vi "Initialize_Labjacks.vi"() -> (0 "error out":errorcluster, 3 "LJ Handles":i32[](array[numeric])=[546668496, 310679472, 546668496])   [LabVIEW 2016]
uses:
  Globals/LJ_Handles_Global.vi
panel:
  in  "Num Devices":i32=3
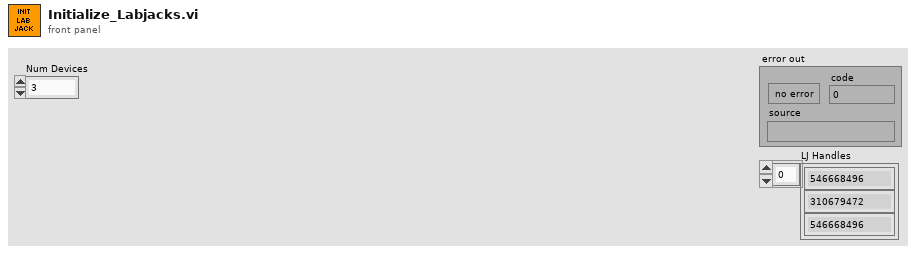
[diagram p1: front panel]
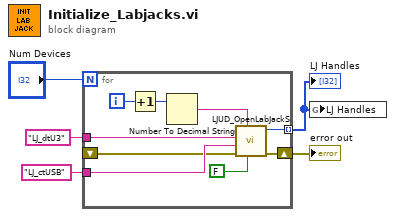
[diagram p0: block diagram]
diagram:
  n1 = for {
    N: "Num Devices" -> [_]
    tunnel: "LJ_dtU3" ("DeviceType") -> [w11]
    tunnel: "LJ_ctUSB" ("ConnectionType") -> [w10]
    tunnel: [w8] -> w1 mode=indexing
    shift-right: [w7] -> w2
    shift-left: _ -> [w6]
    i -> [w14]
    n2 = Increment(x=w14) -> (x+1=w13:i32)
    n3 = Number To Decimal String(number=w13) -> (decimal integer string=w12:string)  [unwired: 1 in]
    n4 = call "LJUD_OpenLabJackS.vi"("FirstFound"=FALSE, "Address"=w12, "error in"=w6, "ConnectionType"=w10, "DeviceType"=w11) -> ("error out"=w7:errorcluster, "Handle"=w8:i32)  [unwired: 4 in, 1 out]
  }
  "error out" <- w2
  "LJ Handles" <- w1
  n5 = global write "LJ_Handles_Global.vi" "LJ Handles"(w1) -> ()
